vi "SVPO Order Metrics for Periodic Inspection (1 Ch) with IC.vi"(0 "even-angle signal":cluster{"r0":dbl, "dr":dbl, "Y":dbl[]}={"r0"=0.0, "dr"=1.0, "Y"=[]} {"r0" format="%.2p"; "dr" format="%.2p"; "Y" format="%.2f"}, 1 "update? (T)":bool=TRUE, 2 "reset? (F)":bool, 7 "even-angle position info":T3, 9 "orders":dbl[](array[numeric])=[1.0] format="%.2f", 11 "integration cycles":u32=8, 12 "measurement selection":T2={"speed"=TRUE, "DC gap"=TRUE, "RMS level"=TRUE, "max-min level"=TRUE, "magnitude"=TRUE, "phase"=TRUE}, 13 "initial conditions":T1) -> (3 "speed [RPM]":dbl, 4 "DC gap":dbl, 6 "RMS level":dbl, 8 "max-min level":dbl, 10 "magnitudes [RMS]":dbl[](array[numeric]), 14 "final conditions":T1, 15 "phase [phase lag]":dbl[](array[numeric]))   [LabVIEW 2017, in "SoundVib_OrderTracking.lvlib"]
doc: "Computes the metrics of designated orders in an even-angle signal, such as magnitudes, phases, speed, DC gap, RMS level, and max-min level. This VI calculates metrics values from the latest integration cycles of the even-angle signal. Use this VI on embedded targets that have limited computational resources. Wire data to the <B>even-angle signal</B> input to determine the polymorphic instance to use or manually select the instance."
uses:
  <vilib>/addons/Sound and Vibration/Order Analysis/Resample Order Tracking/SoundVib_OrderTracking.lvlib
  <vilib>/addons/Sound and Vibration/Order Analysis/Misc/OAT Position Info.ctl
  <vilib>/addons/_NISVFA/_Shared subVIs/Controls/svc_Order Metrics State.ctl
  <vilib>/Analysis/baseanly.llb/Mean (DBL).vi
  <vilib>/Analysis/5stat.llb/RMS (DBL).vi
  <vilib>/Analysis/NI_AALPro.lvlib
  <vilib>/Analysis/NI_AALBase.lvlib
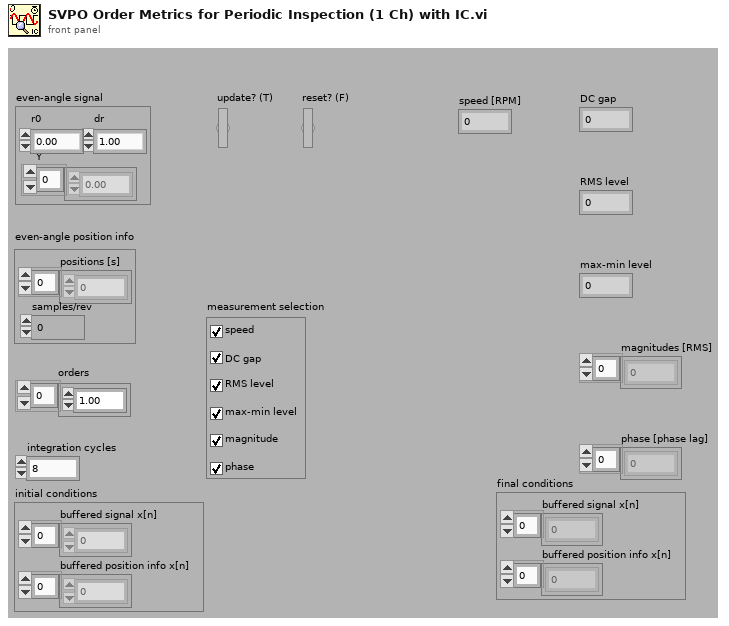
[diagram p1: front panel]
types:
  T1 = typedef "svc_Order Metrics State.ctl" = cluster{"buffered signal x[n]":dbl[], "buffered position info x[n]":dbl[]}
  T2 = cluster{"speed":bool, "DC gap":bool, "RMS level":bool, "max-min level":bool, "magnitude":bool, "phase":bool}
  T3 = typedef "OAT Position Info.ctl" = cluster{"positions [s]":dbl[], "samples/rev":dbl}
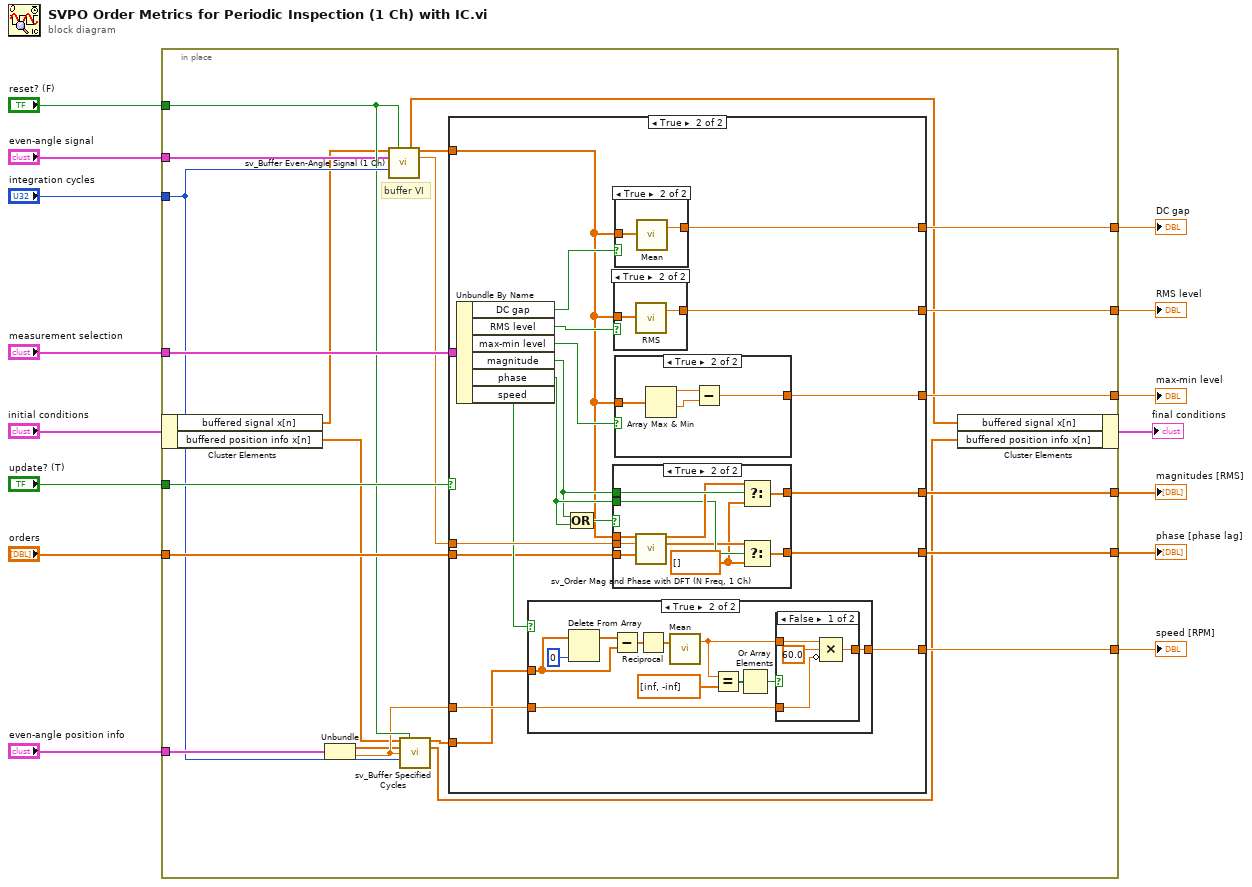
[diagram p0: block diagram]
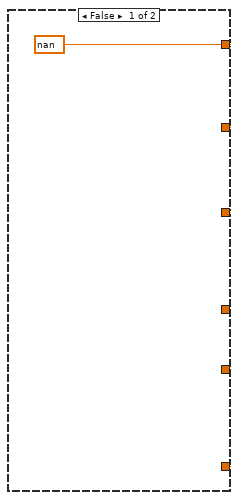
[diagram p2: hidden frame]
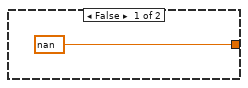
[diagram p3: hidden frame]
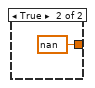
[diagram p4: hidden frame]
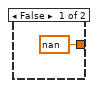
[diagram p5: hidden frame]
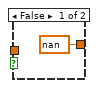
[diagram p7: hidden frame]
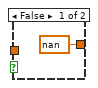
[diagram p8: hidden frame]
diagram:
  n1 = in-place {
    in-place-border: "measurement selection" -> [w37]
    in-place-border: [w36] -> w14
    in-place-border: [w35] -> w13
    in-place-border: "orders" -> [w34]
    in-place-border: [w32] -> w11
    in-place-border: [w31] -> w10
    in-place-border: [w30] -> w9
    in-place-border: "update? (T)" -> [w29]
    in-place-border: "even-angle signal" -> [w19]
    in-place-border: [w27] -> w6
    in-place-border: "even-angle position info" -> [w26]
    in-place-border: "integration cycles" -> [w24]
    in-place-border: "reset? (F)" -> [w23]
    # "buffer VI"
    n2 = in-place-cluster #1("initial conditions") -> ("buffered signal x[n]"=w18:dbl[], "buffered position info x[n]"=w20:dbl[])
    n3 = Unbundle(w26) -> ("positions [s]"=w21:dbl[], "samples/rev"=w22:dbl)
    n4 = call <vilib>:"sv_Buffer Even-Angle Signal (1 Ch).vi"("initial buffered x[n]"=w18, "reset? (True)"=w23, "even-angle signal"=w19, "integration cycles"=w24) -> ("buffered x[n]"=w17:dbl[], "buffered x[n] for analysis"=w33:dbl[], "sample rate"=w28:dbl)  [unwired: 9 in]
    n5 = call <vilib>:"sv_Buffer Specified Cycles.vi"("inital buffered x[n]"=w20, "reset? (True)"=w23, "x[n]"=w21, "fs"=w22, "integration cycles"=w24) -> ("buffered x[n] for analysis"=w25:dbl[], "buffered x[n]"=w16:dbl[])  [unwired: 9 in]
    n6 = case shown="True" w29 {
      tunnel: w37 -> [_ w57]
      tunnel: [w38 w55] -> w36
      tunnel: [w38 w53] -> w35
      tunnel: w34 -> [_ w41]
      tunnel: w28 -> [_ w51]
      tunnel: w33 -> [_ w39]
      tunnel: [_ w49] -> w32
      tunnel: [_ w48] -> w31
      tunnel: [w38 w42] -> w30
      tunnel: [w38 w45] -> w27
      tunnel: w25 -> [_ w40]
      tunnel: w22 -> [_ w43]
      frame False {
        w38 = nan ("mean")
      }
      frame True {
        n7 = Unbundle By Name(w57) -> ("DC gap"=w56:bool, "RMS level"=w54:bool, "max-min level"=w46:bool, "magnitude"=w47:bool, "phase"=w50:bool, "speed"=w44:bool)
        n8 = case shown="True" w44 {
          tunnel: w40 -> [_ w67]
          tunnel: [nan w68] -> w42
          tunnel: w43 -> [_ w64]
          frame False {
          }
          frame True {
            n9 = Delete From Array(array=w67, index=0) -> (array with subset deleted=w59:dbl[])  [unwired: 1 in, 1 out]
            n10 = Subtract(x=w59, y=w67) -> (x-y=w66:dbl[])
            n11 = Reciprocal(x=w66) -> (1/x=w65:dbl[])
            n12 = call-poly <vilib>:"Mean.vi"("X"=w65) -> ("mean"=w63:dbl)  [unwired: 1 out]
            n13 = Equal?(x=w63, y=dbl[] [inf, -inf]) -> (x = y?=w61:bool[])
            n14 = Or Array Elements(Boolean array=w61) -> (logical OR=w60:bool)
            n15 = case shown="False" w60 {
              tunnel: w63 -> [w73 _]
              tunnel: [w71 nan] -> w68
              tunnel: w64 -> [w70 _]
              frame False {
                n16 = Compound Arithmetic op=MULTIPLY(w73, 60.0 ("y"), invert w70) -> (w71:dbl)
              }
              frame True {
              }
            }
          }
        }
        n17 = Compound Arithmetic op=OR(w47, w50) -> (w52:bool)
        n18 = case shown="True" w52 {
          tunnel: w41 -> [_ w89]
          tunnel: w51 -> [_ w88]
          tunnel: w39 -> [_ w87]
          tunnel: w47 -> [_ w86]
          tunnel: w50 -> [_ w84]
          tunnel: [_ w81] -> w49
          tunnel: [_ w80] -> w48
          frame False {
          }
          frame True {
            w82 = dbl[] [] ("f")
            n19 = call <vilib>:"sv_Order Mag and Phase with DFT (N Freq, 1 Ch).vi"("buffered x[n]"=w87, "fs"=w88, "fc [Hz]"=w89) -> ("mag [RMS]"=w85:dbl[], "phase"=w83:dbl[])  [unwired: 11 in]
            n20 = Select(t=w85, s=w86, f=w82) -> (s? t:f=w81:dbl[])
            n21 = Select(t=w83, s=w84, f=w82) -> (s? t:f=w80:dbl[])
          }
        }
        n22 = case shown="True" w54 {
          tunnel: w39 -> [_ w92]
          tunnel: [nan ("mean") w91] -> w53
          frame False {
          }
          frame True {
            n23 = call-poly <vilib>:"RMS.vi"("X"=w92) -> ("rms value"=w91:dbl)  [unwired: 1 out]
          }
        }
        n24 = case shown="True" w56 {
          tunnel: w39 -> [_ w95]
          tunnel: [nan ("mean") w94] -> w55
          frame False {
          }
          frame True {
            n25 = call-poly <vilib>:"Mean.vi"("X"=w95) -> ("mean"=w94:dbl)  [unwired: 1 out]
          }
        }
        n26 = case shown="True" w46 {
          tunnel: w39 -> [_ w79]
          tunnel: [nan w76] -> w45
          frame False {
          }
          frame True {
            n27 = Array Max & Min(array=w79) -> (max value=w78:dbl, min value=w77:dbl)  [unwired: 2 out]
            n28 = Subtract(x=w78, y=w77) -> (x-y=w76:dbl)
          }
        }
      }
    }
    n29 = in-place-cluster #1("buffered signal x[n]"=w17, "buffered position info x[n]"=w16) -> (→"final conditions":T1)
  }
  "magnitudes [RMS]" <- w11
  "phase [phase lag]" <- w10
  "speed [RPM]" <- w9
  "DC gap" <- w14
  "RMS level" <- w13
  "max-min level" <- w6
